vi "strain_test3.vi"() -> ()   [LabVIEW 2014]
uses:
  <vilib>/LabVIEW Targets/FPGA/cRIO/shared/nicrio_ModuleControls/nicrio_cRIO-9237_DataRatesRing.ctl
  <vilib>/LabVIEW Targets/FPGA/cRIO/shared/nicrio_ModuleControls/nicrio_cRIO-9237_ExcitationVoltageRing.ctl
  <vilib>/rvi/Emulation/niFpgaGetClockAttributes.vi
  <vilib>/rvi/Emulation/niFpgaSctlEmulationGetInTimedLoop.vi
  <vilib>/rvi/Emulation/niFpgaEmulationReportErrorSimple.vi
  <vilib>/rvi/eio/common/nirviEmuTemplatePropertySet_errors.vi
  <vilib>/rvi/eio/common/nirviEmuTemplateMethod_errors.vi
  <vilib>/rvi/Emulation/niFpgaCriticalErrorInLSC.vi
  <vilib>/eio/EIOPropertyNode/EIOPropertyNode.xnode
  <vilib>/eio/EIONode/EIONode.xnode
  <vilib>/rvi/Analysis/measure/butterworth/XNode/niFpgaButterworthFilter.xnode
  <vilib>/rvi/eio/common/nirviEmuTemplatePropertyGet_errors.vi
  <vilib>/rvi/eio/common/nirviEmuTemplatePropertyGet_noerrors.vi
  <vilib>/rvi/eio/common/nirviEmuTemplatePropertySet_noerrors.vi
panel:
  in  "Reset":bool
  in  "Stop":bool
  out "Force":fxp<+/-,64,27>
  out "Raw Force":fxp<+/-,64,23>
  in  "S/F coeff":fxp<+/-,40,15>
  out "Strain":fxp<+/-,48,2>
  out "Raw Strain":fxp<+/-,44,-2>
  out "Filtered data":fxp<+/-,28,0>
  out "Mod6/AI2":fxp<+/-,24,-4>
  in  "Excitation Voltage":T1 items=["2.5 Volts", "3.3 Volts", "5.0 Volts", "10.0 Volts", "External Excitation"]
  in  "Data Rate":T2=1 items=["50.000 kS/s (NI 9237)"=1, "25.000 kS/s (NI 9237)"=2, "16.667 kS/s (NI 9237)"=3, "12.500 kS/s (NI 9237)"=4, "10.000 kS/s (NI 9237)"=5, "8.333 kS/s (NI 9237)"=6, "7.143 kS/s (NI 9237)"=7, "6.250 kS/s (NI 9237)"=8, "5.556 kS/s (NI 9237)"=9, "5.000 kS/s (NI 9237)"=10, "4.545 kS/s (NI 9237)"=11, "4.167 kS/s (NI 9237)"=12, "3.846 kS/s (NI 9237)"=13, "3.571 kS/s (NI 9237)"=14, "3.333 kS/s (NI 9237)"=15, "3.125 kS/s (NI 9237)"=16, "2.941 kS/s (NI 9237)"=17, "2.778 kS/s (NI 9237)"=18, "2.632 kS/s (NI 9237)"=19, "2.500 kS/s (NI 9237)"=20, "2.381 kS/s (NI 9237)"=21, "2.273 kS/s (NI 9237)"=22, "2.174 kS/s (NI 9237)"=23, "2.083 kS/s (NI 9237)"=24, "2.000 kS/s (NI 9237)"=25, "1.923 kS/s (NI 9237)"=26, "1.852 kS/s (NI 9237)"=27, "1.786 kS/s (NI 9237)"=28, "1.724 kS/s (NI 9237)"=29, "1.667 kS/s (NI 9237)"=30, "1.613 kS/s (NI 9237)"=31]
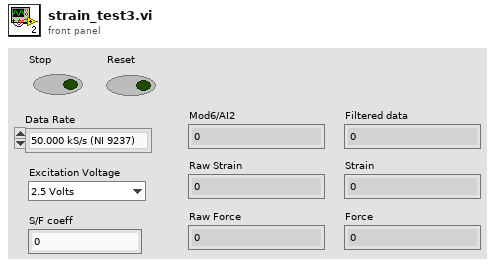
[diagram p1: front panel]
types:
  T1 = typedef "nicrio_cRIO-9237_ExcitationVoltageRing.ctl" = u8
  T2 = typedef "nicrio_cRIO-9237_DataRatesRing.ctl" = u8
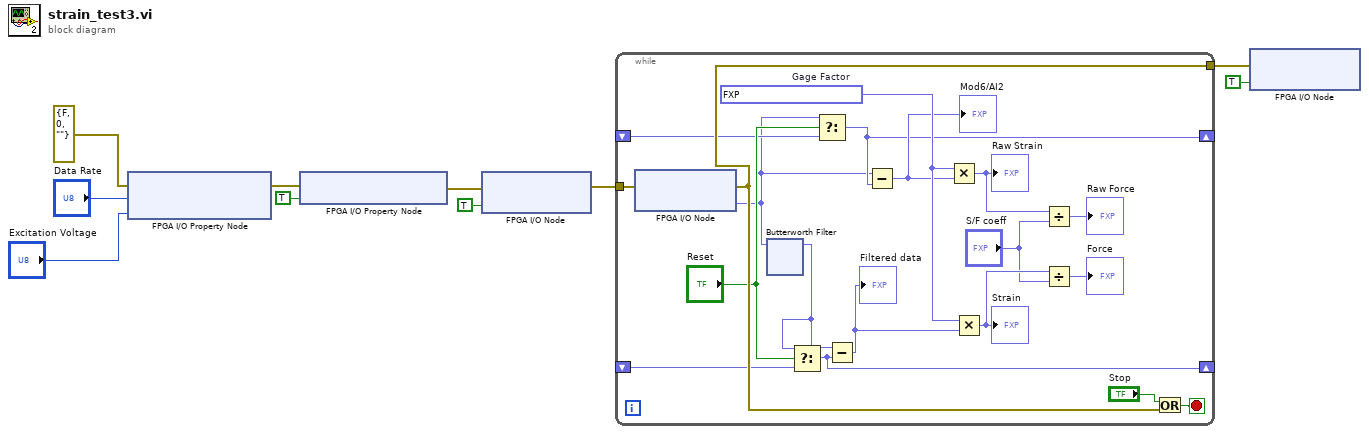
[diagram p0: block diagram]
diagram:
  n1 = xnode "FPGA I/O Property Node"("error in"=errorcluster {"status"=FALSE, "code"=0, "source"=""}, "Data Rate"="Data Rate", "Excitation Voltage"="Excitation Voltage") -> ("error out"=w10:errorcluster)  [unwired: 1 in, 1 out]
  n2 = xnode "FPGA I/O Property Node"("error in"=w10, "Half-Bridge Enable"=TRUE) -> ("error out"=w5:errorcluster)  [unwired: 1 in, 1 out]
  n3 = xnode "FPGA I/O Node"("error in"=w5, "Mod6/Start"=TRUE) -> ("error out"=w3:errorcluster)  [unwired: 1 in, 1 out]
  n4 = while {
    tunnel: w3 -> [w29]
    tunnel: [w21] -> w2
    shift-right: [w18] -> _
    shift-left: _ -> [w20]
    shift-right: [w13] -> _
    shift-left: _ -> [w15]
    stop <- w12 stop-if-true
    w28 = fxp<+,20,2> 2.115001678466797  # Gage Factor
    n5 = xnode "FPGA I/O Node"("error in"=w29) -> ("error out"=w21:errorcluster, "Mod6/AI2"=w11:fxp<+/-,24,-4>)  [unwired: 1 in, 1 out]
    n6 = xnode "Butterworth Filter"("input data"=w11) -> ("output data"=w19:fxp<+/-,28,0>)  [unwired: 2 in]
    n7 = Select(t=w19, s="Reset", f=w20) -> (s? t:f=w18:fxp<+/-,28,0>)
    n8 = Select(t=w11, s="Reset", f=w15) -> (s? t:f=w13:fxp<+/-,24,-4>)
    n9 = Subtract(x=w19, y=w18) -> (x-y=w17:fxp<+/-,32,16>)
    "Filtered data" <- w17
    n10 = Subtract(x=w11, y=w13) -> (x-y=w14:fxp<+/-,32,16>)
    "Mod6/AI2" <- w14
    n11 = Multiply(x=w28, y=w14) -> (x*y=w27:fxp<+/-,52,18>)
    "Raw Strain" <- w27
    n12 = Multiply(x=w28, y=w17) -> (x*y=w25:fxp<+/-,52,18>)
    "Strain" <- w25
    n13 = Divide(x=w27, y="S/F coeff") -> (x/y=→"Raw Force":fxp<+/-,64,43>)
    n14 = Divide(x=w25, y="S/F coeff") -> (x/y=→"Force":fxp<+/-,64,43>)
    n15 = Or(x="Stop", y=w21) -> (x .or. y?=w12:bool)
  }
  n16 = xnode "FPGA I/O Node"("error in"=w2, "Mod6/Stop"=TRUE) -> ()  [unwired: 1 in, 2 out]
